vi "Parse Array.vi"(8 "error in (no error)":errorcluster, 10 "Index In":i32, 11 "JSON String":string) -> (0 "error out":errorcluster, 2 "Index Out":i32, 3 "JSON Value out":variant)   [LabVIEW 2017, in "Advanced Variant Tools.lvlib" / "JSON Support.lvlib"]
uses:
  JSON Support.lvlib
  Errors.ctl
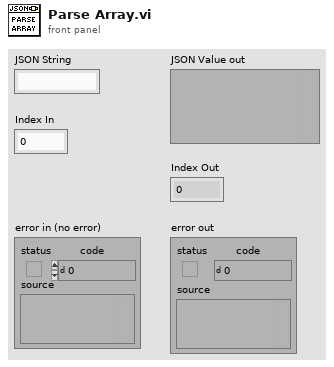
[diagram p1: front panel]
types:
  T1 = typedef "Advanced Variant Tools.lvlib/JSON Support.lvlib/Errors.ctl" = enum16{"No key", "Key path type", "Array OOB", "Type Mismatch", "Invalid Token", "Invalid Value"}
  T2 = typedef "Advanced Variant Tools.lvlib/JSON Support.lvlib/Token Type.ctl" = enum16{"NONE", "CURLY_OPEN", "CURLY_CLOSE", "SQUARED_OPEN", "SQUARED_CLOSE", "COLON", "COMMA", "STRING", "NUMBER", "TRUE", "FALSE", "NULL"}
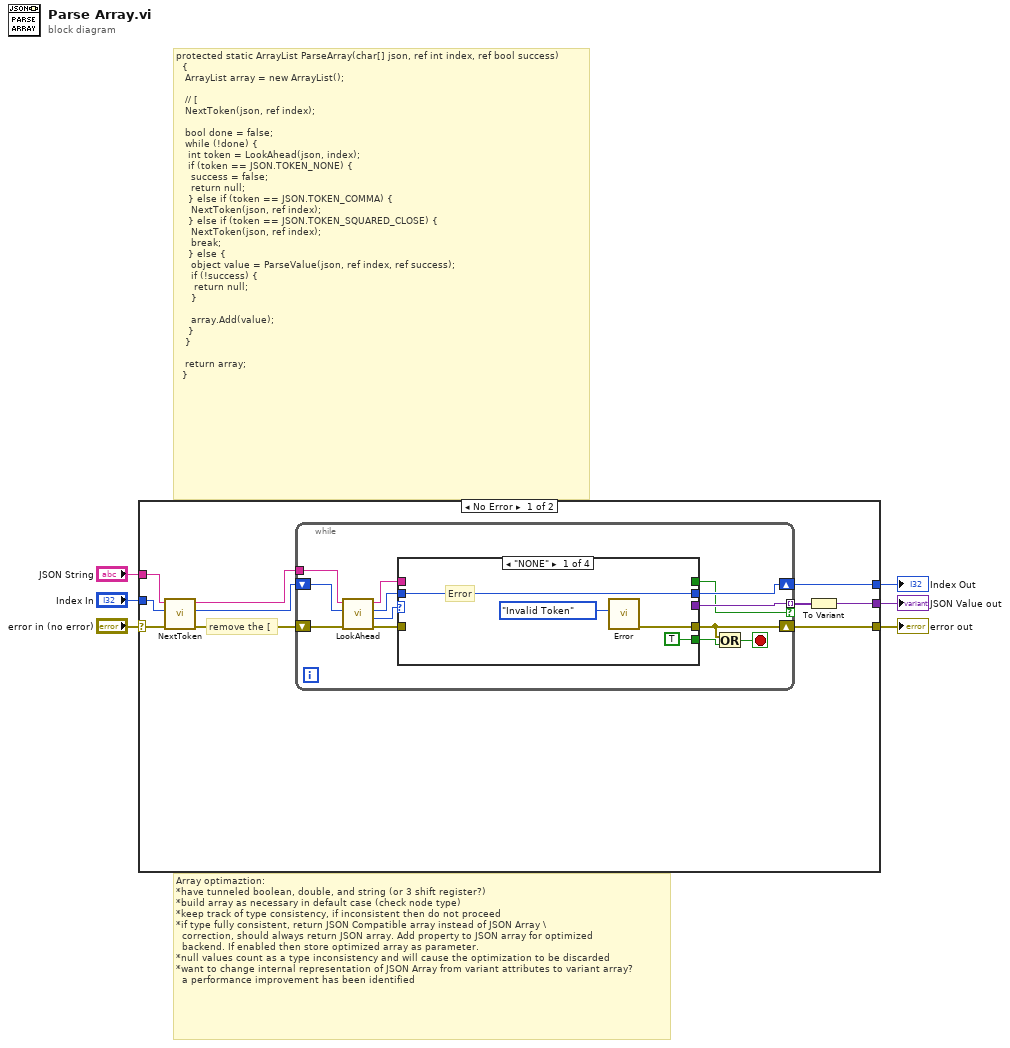
[diagram p0: block diagram]
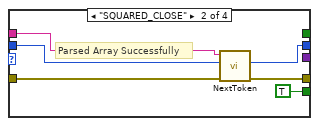
[diagram p2: hidden frame]
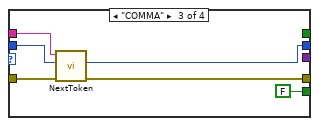
[diagram p3: hidden frame]
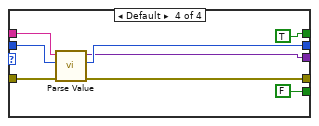
[diagram p4: hidden frame]
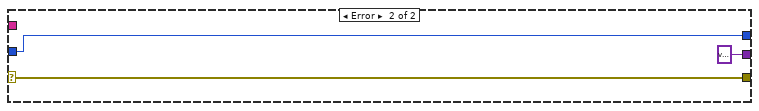
[diagram p5: hidden frame]
diagram:
  # "Array optimaztion:\n*have tunneled boolean, double, and string (or 3 shift register?)\n*build array as necessary in default case (check node type)\n*keep track of type consistency, if inconsistent then do not proceed\n*if type fully consistent, return JSON Compatible array instead of JSON Array \\\n  correction, should always return JSON array. Add property to JSON array for optimized\n  backend. If enabled then store optimized array as parameter.\n*null values count as a type inconsistency and will cause the optimization to be discarded\n*want to change internal representation of JSON Array from variant attributes to variant array?\n  a performance improvement has been identified"
  # "protected static ArrayList ParseArray(char[] json, ref int index, ref bool success)\n\t\t{\n\t\t\tArrayList array = new ArrayList();\n\n\t\t\t// [\n\t\t\tNextToken(json, ref index);\n\n\t\t\tbool done = false;\n\t\t\twhile (!done) {\n\t\t\t\tint token = LookAhead(json, index);\n\t\t\t\tif (token == JSON.TOKEN_NONE) {\n\t\t\t\t\tsuccess = false;\n\t\t\t\t\treturn null;\n\t\t\t\t} else if (token == JSON.TOKEN_COMMA) {\n\t\t\t\t\tNextToken(json, ref index);\n\t\t\t\t} else if (token == JSON.TOKEN_SQUARED_CLOSE) {\n\t\t\t\t\tNextToken(json, ref index);\n\t\t\t\t\tbreak;\n\t\t\t\t} else {\n\t\t\t\t\tobject value = ParseValue(json, ref index, ref success);\n\t\t\t\t\tif (!success) {\n\t\t\t\t\t\treturn null;\n\t\t\t\t\t}\n\n\t\t\t\t\tarray.Add(value);\n\t\t\t\t}\n\t\t\t}\n\n\t\t\treturn array;\n\t\t}"
  n1 = case shown="No Error" "error in (no error)" {
    selector: "error in (no error)" -> [w16 w55]
    tunnel: [w8 w55] -> w5
    tunnel: "Index In" -> [w15 w56]
    tunnel: [w11 w56] -> w3
    tunnel: [w7 variant] -> w1
    tunnel: "JSON String" -> [w10 _]
    frame No Error {
      # "remove the ["
      n2 = call "NextToken.vi"("error in (no error)"=w16, "Index In"=w15, "JSON String"=w10) -> ("error out"=w12:errorcluster, "Index Out"=w14:i32, "JSON String Passthrough"=w13:string)  [unwired: 5 in, 1 out]
      n3 = while {
        shift-right: [w22] -> w11
        shift-left: w14 -> [w28]
        tunnel: w13 -> [w27]
        shift-right: [w19] -> w8
        shift-left: w12 -> [w29]
        tunnel: [w18] -> w9 mode=indexing if=w17
        stop <- w20 stop-if-true
        n4 = call "LookAhead.vi"("error in (no error)"=w29, "Index"=w28, "JSON String"=w27) -> ("error out"=w25:errorcluster, "TOKEN"=w26:T2, "Index Passthrough"=w24:i32, "JSON String Passthrough"=w23:string)  [unwired: 5 in]
        n5 = case shown="\"NONE\"" w26 {
          tunnel: w25 -> [_ w39 w43 w53]
          tunnel: [TRUE TRUE FALSE FALSE] -> w21
          tunnel: w24 -> [w32 w38 w44 w52]
          tunnel: w23 -> [_ w37 w45 w51]
          tunnel: [w32 w35 w41 w50] -> w22
          tunnel: [w31 w36 w42 w48] -> w19
          tunnel: [_ _ _ w47] -> w18
          tunnel: [_ _ _ TRUE] -> w17
          frame "NONE" {
            # "Error"
            n6 = call "Error.vi"(9:Errors."Invalid Token") -> ("error out"=w31:errorcluster)  [unwired: 9 in]
          }
          frame "SQUARED_CLOSE" {
            # "Parsed Array Successfully"
            n7 = call "NextToken.vi"("error in (no error)"=w39, "Index In"=w38, "JSON String"=w37) -> ("error out"=w36:errorcluster, "Index Out"=w35:i32)  [unwired: 5 in, 2 out]
          }
          frame "COMMA" {
            n8 = call "NextToken.vi"("error in (no error)"=w43, "Index In"=w44, "JSON String"=w45) -> ("error out"=w42:errorcluster, "Index Out"=w41:i32)  [unwired: 5 in, 2 out]
          }
          frame Default {
            n9 = call "Parse Value.vi"("error in (no error)"=w53, "Index In"=w52, "JSON String"=w51) -> ("error out"=w48:errorcluster, "Index Out"=w50:i32, "JSON Value out"=w47:variant)  [unwired: 6 in]
          }
        }
        n10 = Or(x=w19, y=w21) -> (x .or. y?=w20:bool)
      }
      n11 = To Variant(anything=w9) -> (Variant=w7:variant)
    }
    frame Error {
    }
  }
  "error out" <- w5
  "Index Out" <- w3
  "JSON Value out" <- w1
